vi "NI-XNET RT Driver VI.vi"(7 "Operation":T4, 11 "Device Reference in":T5 format="%.0x") -> (0 "Error Code":i32)   [LabVIEW 2009, in "NI-XNET Custom Device.lvlib"]
uses:
  NI-XNET Custom Device.lvlib
  <vilib>/NI VeriStand/Custom Device API/Custom Device Item Ref.ctl
  <vilib>/NI VeriStand/Custom Device API/Hardware Interface Driver VI Operation.ctl
  <vilib>/NI VeriStand/Custom Device API/Data Reference.ctl
  <vilib>/NI VeriStand/Custom Device API/Block Data Reference.ctl
  <vilib>/xnet/xnet.llb/XNET String To IO Name (Interface).vi
  <vilib>/NI VeriStand/Custom Device API/Get Item Property (String).vi
  <vilib>/xnet/xnet.llb/XNET Create Session (Signal Input Single-point).vi
  <vilib>/xnet/xnet.llb/XNET Read (Signal Single-point).vi
  <vilib>/xnet/xnet.llb/XNET Control Scope.ctl
  <vilib>/xnet/xnet.llb/XNET Write (Signal Single-point).vi
  <vilib>/NI VeriStand/Custom Device API/Custom Device API.lvlib
panel:
  in  "cluster":T3 {"Input Data Refs"."Data Reference" format="%.0x"; "Output Data Refs"."Data Reference" format="%.0x"; "Output Enable Refs" format="%.0x"}
  # "Items used for output sessions\nand enable/disable functionality"
  # "Veristand custom device items"
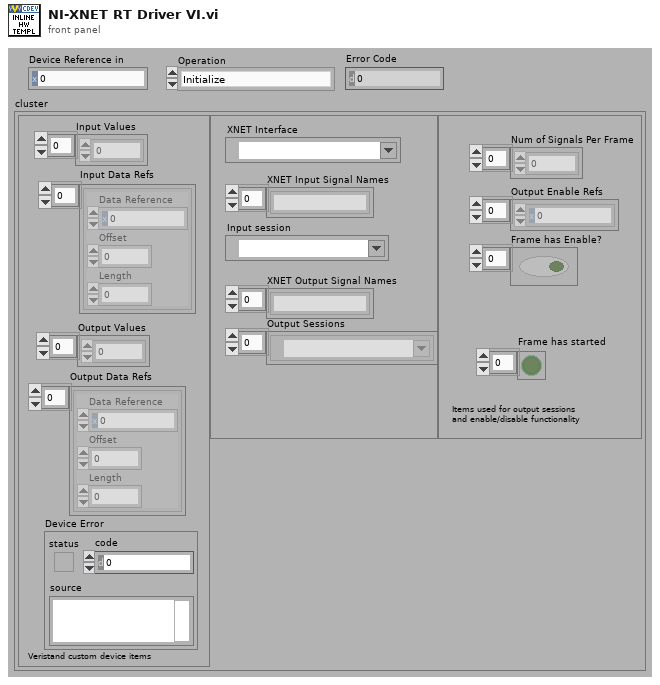
[diagram p1: front panel]
types:
  T1 = typedef "Custom Device API.lvlib/Data Reference.ctl" = i32
  T2 = typedef "Custom Device API.lvlib/Block Data Reference.ctl" = cluster{"Data Reference":T1, "Offset":i32, "Length":i32}
  T3 = cluster{"Input Values":dbl[], "Output Values":dbl[], "Device Error":errorcluster, "XNET Interface":refnum<k21>, "XNET Input Signal Names":string[], "Input session":refnum<k21>, "XNET Output Signal Names":string[], "Output Sessions":refnum<k21>[], "Num of Signals Per Frame":i32[], "Output Enable Refs":T1[], "Frame has Enable?":bool[], "Output Data Refs":T2[], "Input Data Refs":T2[], "Frame has started":bool[]}
  T4 = typedef "Custom Device API.lvlib/Hardware Interface Driver VI Operation.ctl" = enum16{"Initialize", "Start", "Read Data from HW", "Write Data to HW", "Close"}
  T5 = typedef "Custom Device API.lvlib/Custom Device Item Ref.ctl" = u64
  T6 = typedef "XNET Control Scope.ctl" = u32
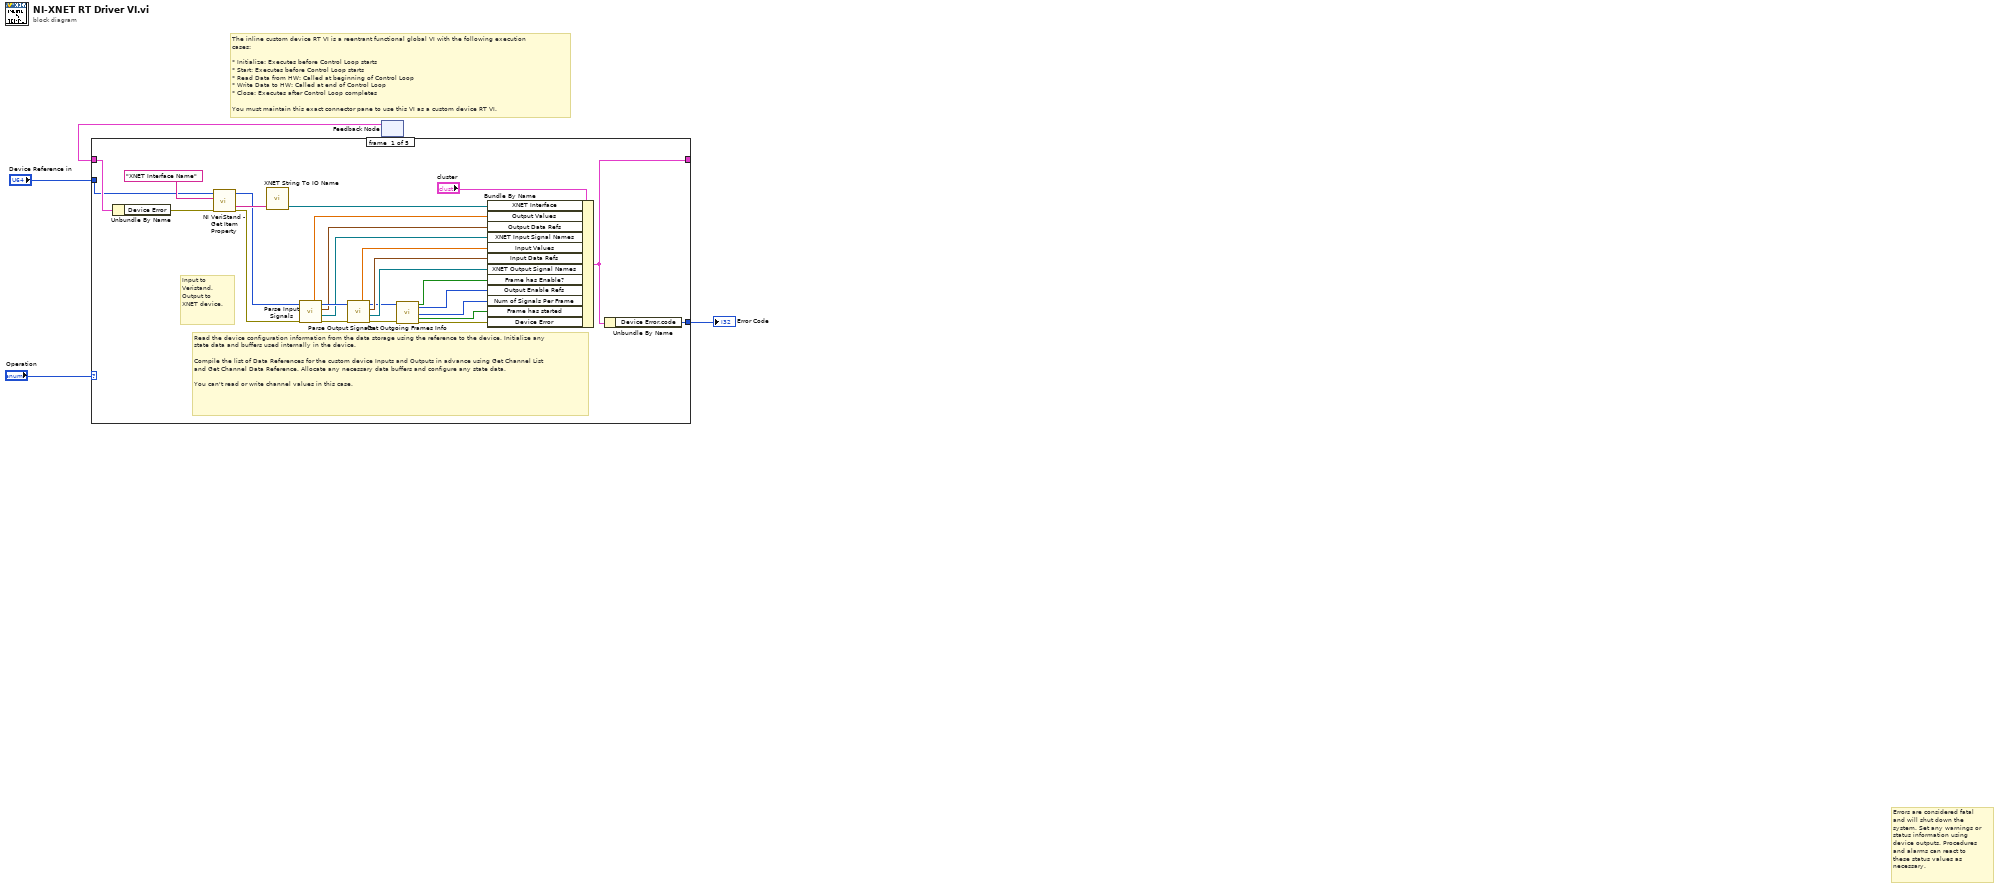
[diagram p0: block diagram]
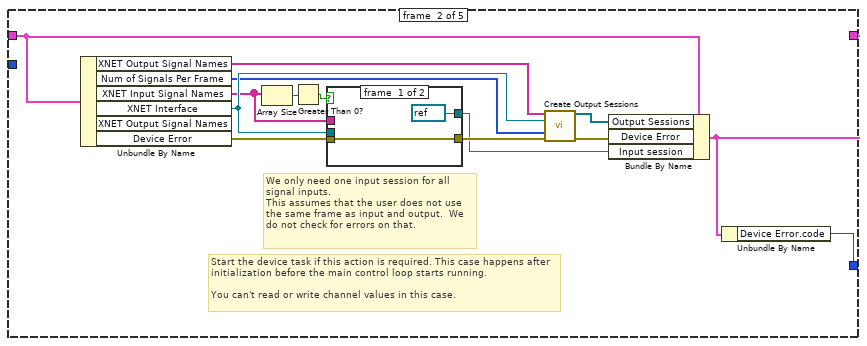
[diagram p2: hidden frame]
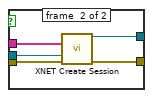
[diagram p3: hidden frame]
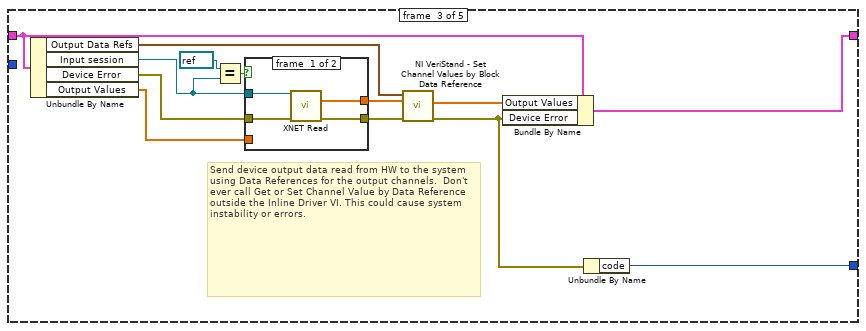
[diagram p4: hidden frame]
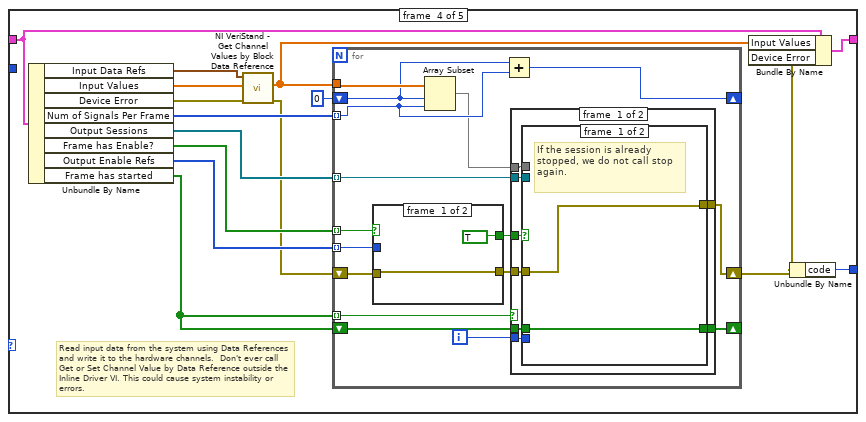
[diagram p6: hidden frame]
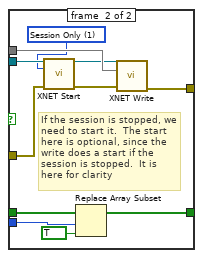
[diagram p7: hidden frame]
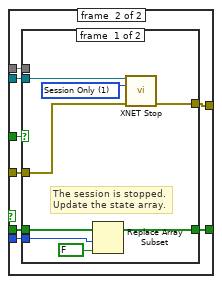
[diagram p8: hidden frame]
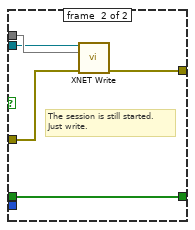
[diagram p9: hidden frame]
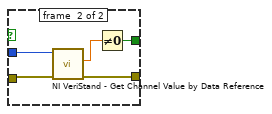
[diagram p10: hidden frame]
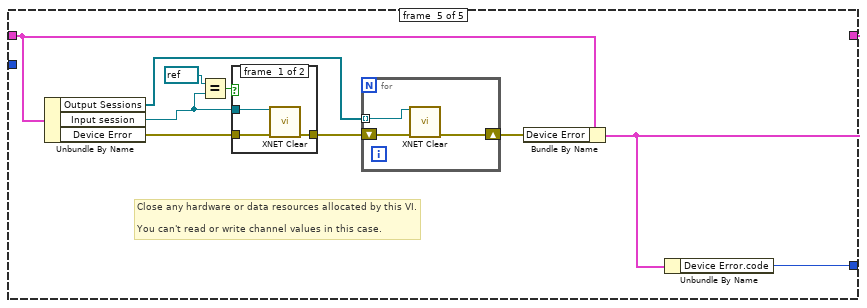
[diagram p11: hidden frame]
diagram:
  # "Errors are considered fatal and will shut down the system. Set any warnings or status information using device outputs. Procedures and alarms can react to these status values as necessary."
  # "The inline custom device RT VI is a reentrant functional global VI with the following execution cases:\n\n* Initialize: Executes before Control Loop starts\n* Start: Executes before Control Loop starts\n* Read Data from HW: Called at beginning of Control Loop\n* Write Data to HW: Called at end of Control Loop\n* Close: Executes after Control Loop completes\n\nYou must maintain this exact connector pane to use this VI as a custom device RT VI."
  n1 = feedback #1() -> (w3:T3)  [unwired: 1 out]
  n2 = case shown="\"Close\"" "Operation" {
    tunnel: [w7 w44 w64 w85 w159] -> w4
    tunnel: w3 -> [w23 w45 w63 w86 w160]
    tunnel: "Device Reference in" -> [w22 _ _ _ _]
    tunnel: [w28 w43 w65 w84 w161] -> w1
    frame #0 {
      # "Read the device configuration information from the data storage using the reference to the device. Initialize any state data and buffers used internally in the device.\n\nCompile the list of Data References for the custom device Inputs and Outputs in advance using Get Channel List and Get Channel Data Reference. Allocate any necessary data buffers and configure any state data.\n\nYou can't read or write channel values in this case."
      # "Input to Veristand.  Output to XNET device."
      n3 = Unbundle By Name(w23) -> ("Device Error"=w16:errorcluster)
      n4 = call-poly <vilib>:"NI VeriStand - Get Item Property.vi"("error in (no error)"=w16, "Property Name"="XNET Interface Name", "Item Ref in"=w22) -> ("error out"=w15:errorcluster, "Value"=w30:string, "Item Ref out"=w10:T5)  [unwired: 5 in, 1 out]
      n5 = call-poly <vilib>:"XNET String To IO Name.vi"("string"=w30) -> ("XNET Interface"=w27:refnum<k21>)  [unwired: 4 in]
      n6 = call "Parse Input Signals.vi"("error in (no error)"=w15, "Device Reference in"=w10) -> ("error out"=w19:errorcluster, "Input Signals"=w17:refnum<k21>[], "Block Data Refs"=w18:T2[], "Device Ref out"=w20:T5, "Output Values"=w21:dbl[])  [unwired: 5 in]
      n7 = call "Parse Output Signals.vi"("error in (no error)"=w19, "Device Ref in"=w20) -> ("error out"=w8:errorcluster, "XNET Output Signal Names"=w26:refnum<k21>[], "Input Data Refs"=w25:T2[], "Device Ref out"=w9:T5, "Input Values"=w24:dbl[])  [unwired: 5 in]
      n8 = call "Get Outgoing Frames Info.vi"("Device Reference in"=w9, "error in (no error)"=w8) -> ("Enable Present?"=w13:bool[], "Enable Refs"=w12:T1[], "Number of Signals Per Frame"=w11:i32[], "Started?"=w6:bool[], "error out"=w14:errorcluster)  [unwired: 13 in]
      n9 = Bundle By Name(cluster="cluster", "XNET Interface"=w27, "Output Values"=w21, "Output Data Refs"=w18, "XNET Input Signal Names"=w17, "Input Values"=w24, "Input Data Refs"=w25, "XNET Output Signal Names"=w26, "Frame has Enable?"=w13, "Output Enable Refs"=w12, "Num of Signals Per Frame"=w11, "Frame has started"=w6, "Device Error"=w14) -> (w7:T3)
      n10 = Unbundle By Name(w7) -> ("Device Error.code"=w28:i32)
    }
    frame #1 {
      # "We only need one input session for all signal inputs.\nThis assumes that the user does not use the same frame as input and output.  We do not check for errors on that."
      # "Start the device task if this action is required. This case happens after initialization before the main control loop starts running.\n\nYou can't read or write channel values in this case."
      n11 = Unbundle By Name(w45) -> ("XNET Output Signal Names"=w39:string[], "Num of Signals Per Frame"=w37:i32[], "XNET Input Signal Names"=w34:string[], "XNET Interface"=w38:refnum<k21>, "Device Error"=w40:errorcluster)  [unwired: 1 out]
      n12 = Array Size(array=w34) -> (size(s)=w33:i32)
      n13 = Greater Than 0?(x=w33) -> (x > 0?=w32:bool)
      n14 = case shown="True" w32 {
        tunnel: [w47 w52] -> w42
        tunnel: w40 -> [w47 w51]
        tunnel: w38 -> [_ w50]
        tunnel: [refnum<k21> refnum ("session out") w49] -> w35
        tunnel: w34 -> [_ w48]
        frame #0 {
        }
        frame #1 {
          n15 = call-poly <vilib>:"XNET Create Session.vi"("signal list"=w48, "interface"=w50, "error in (no error)"=w51) -> ("session out"=w49:refnum<k21>, "error out"=w52:errorcluster)  [unwired: 11 in]
        }
      }
      n16 = call "Create Output Sessions.vi"("XNET Output Signal Names"=w39, "XNET Interface"=w38, "Num of Signals Per Frame"=w37, "error in"=w42) -> ("Output Sessions"=w36:refnum<k21>[], "error out"=w41:errorcluster)  [unwired: 10 in]
      n17 = Bundle By Name(cluster=w45, "Output Sessions"=w36, "Device Error"=w41, "Input session"=w35) -> (w44:T3)
      n18 = Unbundle By Name(w44) -> ("Device Error.code"=w43:i32)
    }
    frame #2 {
      # "Send device output data read from HW to the system using Data References for the output channels.  Don't ever call Get or Set Channel Value by Data Reference outside the Inline Driver VI. This could cause system instability or errors."
      n19 = Unbundle By Name(w63) -> ("Output Data Refs"=w58:T2[], "Input session"=w56:refnum<k21>, "Device Error"=w59:errorcluster, "Output Values"=w53:dbl[])
      n20 = Equal?(x=refnum<k21> refnum ("session out"), y=w56) -> (x = y?=w54:bool)
      n21 = case shown="False" w54 {
        tunnel: [w69 w70] -> w62
        tunnel: [w68 w71] -> w61
        tunnel: w56 -> [w67 _]
        tunnel: w59 -> [w66 w71]
        tunnel: w53 -> [_ w70]
        frame #0 {
          n22 = call-poly <vilib>:"XNET Read.vi"("session in"=w67, "error in (no error)"=w66) -> ("data"=w69:dbl[], "error out"=w68:errorcluster)  [unwired: 11 in, 1 out]
        }
        frame #1 {
        }
      }
      n23 = call <vilib>:"NI VeriStand - Set Channel Values by Block Data Reference.vi"("error in (no error)"=w61, "Values Array in"=w62, "Block Data Ref"=w58) -> ("error out"=w60:errorcluster, "Values Array out"=w57:dbl[])  [unwired: 7 in]
      n24 = Bundle By Name(cluster=w63, "Output Values"=w57, "Device Error"=w60) -> (w64:T3)
      n25 = Unbundle By Name(w60) -> ("code"=w65:i32)
    }
    frame #3 {
      # "Read input data from the system using Data References and write it to the hardware channels.  Don't ever call Get or Set Channel Value by Data Reference outside the Inline Driver VI. This could cause system instability or errors."
      n26 = Unbundle By Name(w86) -> ("Input Data Refs"=w75:T2[], "Input Values"=w76:dbl[], "Device Error"=w77:errorcluster, "Num of Signals Per Frame"=w81:i32[], "Output Sessions"=w80:refnum<k21>[], "Frame has Enable?"=w79:bool[], "Output Enable Refs"=w78:T1[], "Frame has started"=w72:bool[])
      n27 = call <vilib>:"NI VeriStand - Get Channel Values by Block Data Reference.vi"("error in (no error)"=w77, "Values Array in"=w76, "Block Data Ref"=w75) -> ("error out"=w73:errorcluster, "Values Array out"=w74:dbl[])  [unwired: 7 out]
      n28 = for {
        tunnel: w74 -> [w102]
        tunnel: w80 -> [w101] mode=indexing
        tunnel: w81 -> [w99] mode=indexing
        shift-right: [w97] -> _
        shift-left: 0 -> [w100]
        tunnel: w79 -> [w95] mode=indexing
        tunnel: w78 -> [w91] mode=indexing
        shift-right: [w96] -> w82
        shift-left: w73 -> [w93]
        tunnel: w72 -> [w90] mode=indexing
        shift-right: [w89] -> _
        shift-left: w72 -> [w88]
        i -> [w87]
        n29 = case shown="True" w95 {
          tunnel: w91 -> [_ w147]
          tunnel: [TRUE w150] -> w94
          tunnel: w93 -> [w145 w149]
          tunnel: [w145 w148] -> w92
          frame #0 {
          }
          frame #1 {
            n30 = call <vilib>:"NI VeriStand - Get Channel Value by Data Reference.vi"("error in (no error)"=w149, "Data Reference in"=w147) -> ("error out"=w148:errorcluster, "Value"=w151:dbl)  [unwired: 8 out]
            n31 = Not Equal To 0?(x=w151) -> (x != 0?=w150:bool)
          }
        }
        n32 = Array Subset(array=w102, index=w100, length=w99) -> (w98:dbl[])
        n33 = Add(x=w100, y=w99) -> (x+y=w97:i32)
        n34 = case shown="True" w90 {
          tunnel: w101 -> [w108 w131]
          tunnel: w98 -> [w109 w130]
          tunnel: [w106 w129] -> w96
          tunnel: w94 -> [w110 w128]
          tunnel: w92 -> [w107 w127]
          tunnel: [w103 w126] -> w89
          tunnel: w88 -> [w105 w125]
          tunnel: w87 -> [w104 w124]
          frame #0 {
            n35 = case shown="True" w110 {
              tunnel: w108 -> [_ w119]
              tunnel: w109 -> [_ w123]
              tunnel: [w112 w122] -> w106
              tunnel: w107 -> [w112 w117]
              tunnel: w105 -> [w111 w116]
              tunnel: w104 -> [_ w115]
              tunnel: [w111 w113] -> w103
              frame #0 {
                # "If the session is already stopped, we do not call stop again."
              }
              frame #1 {
                w118 = T6 1 items=["Normal", "Session Only", "Interface Only"] ("scope (normal)")
                # "If the session is stopped, we need to start it.  The start here is optional, since the write does a start if the session is stopped.  It is here for clarity"
                n36 = call <vilib>:"XNET Start.vi"("session in"=w119, "scope (normal)"=w118, "error in (no error)"=w117) -> ("session out"=w121:refnum<k21>, "error out"=w120:errorcluster)  [unwired: 11 in]
                n37 = Replace Array Subset(array=w116, new element=TRUE ("new element/subarray"), index=w115) -> (w113:bool[])
                n38 = call-poly <vilib>:"XNET Write.vi"("session in"=w121, "data"=w123, "error in (no error)"=w120) -> ("error out"=w122:errorcluster)  [unwired: 11 in, 1 out]
              }
            }
          }
          frame #1 {
            n39 = case shown="True" w128 {
              tunnel: w131 -> [w137 w141]
              tunnel: w130 -> [_ w144]
              tunnel: [w139 w143] -> w129
              tunnel: w127 -> [w138 w142]
              tunnel: [w132 w140] -> w126
              tunnel: w125 -> [w135 w140]
              tunnel: w124 -> [w133 _]
              frame #0 {
                w136 = T6 1 items=["Normal", "Session Only", "Interface Only"] ("scope (normal)")
                # "The session is stopped.  \nUpdate the state array."
                n40 = Replace Array Subset(array=w135, new element=FALSE ("new element/subarray"), index=w133) -> (w132:bool[])
                n41 = call <vilib>:"XNET Stop.vi"("session in"=w137, "scope (normal)"=w136, "error in (no error)"=w138) -> ("error out"=w139:errorcluster)  [unwired: 11 in, 1 out]
              }
              frame #1 {
                # "The session is still started.\nJust write."
                n42 = call-poly <vilib>:"XNET Write.vi"("session in"=w141, "data"=w144, "error in (no error)"=w142) -> ("error out"=w143:errorcluster)  [unwired: 11 in, 1 out]
              }
            }
          }
        }
      }
      n43 = Bundle By Name(cluster=w86, "Input Values"=w74, "Device Error"=w82) -> (w85:T3)
      n44 = Unbundle By Name(w82) -> ("code"=w84:i32)
    }
    frame #4 {
      # "Close any hardware or data resources allocated by this VI.\n\nYou can't read or write channel values in this case."
      n45 = Unbundle By Name(w160) -> ("Output Sessions"=w156:refnum<k21>[], "Input session"=w152:refnum<k21>, "Device Error"=w155:errorcluster)
      n46 = Equal?(x=refnum<k21> refnum ("session out"), y=w152) -> (x = y?=w153:bool)
      n47 = case shown="True" w153 {
        tunnel: w152 -> [w164 _]
        tunnel: [w163 w165] -> w158
        tunnel: w155 -> [w162 w165]
        frame #0 {
          n48 = call <vilib>:"XNET Clear.vi"("session in"=w164, "error in (no error)"=w162) -> ("error out"=w163:errorcluster)  [unwired: 13 in]
        }
        frame #1 {
        }
      }
      n49 = for {
        tunnel: w156 -> [w168] mode=indexing
        shift-right: [w166] -> w157
        shift-left: w158 -> [w167]
        n50 = call <vilib>:"XNET Clear.vi"("session in"=w168, "error in (no error)"=w167) -> ("error out"=w166:errorcluster)  [unwired: 13 in]
      }
      n51 = Bundle By Name(cluster=w160, "Device Error"=w157) -> (w159:T3)
      n52 = Unbundle By Name(w159) -> ("Device Error.code"=w161:i32)
    }
  }
  "Error Code" <- w1
